vi "parseDataBoolean.vi"(8 "error in (no error)":errorcluster, 10 "Index":i32, 11 "U8ArrayParserManualIndexing in":refnum<class "U8ArrayParserManualIndexing.lvclass">) -> (0 "error out":errorcluster, 1 "Data":bool, 2 "Index out":i32, 3 "U8ArrayParserManualIndexing out":refnum<class "U8ArrayParserManualIndexing.lvclass">)   [LabVIEW 2016, in "RTUtilities.lvlib" / "U8ArrayParserManualIndexing.lvclass"]
uses:
  U8ArrayParserManualIndexing.lvclass
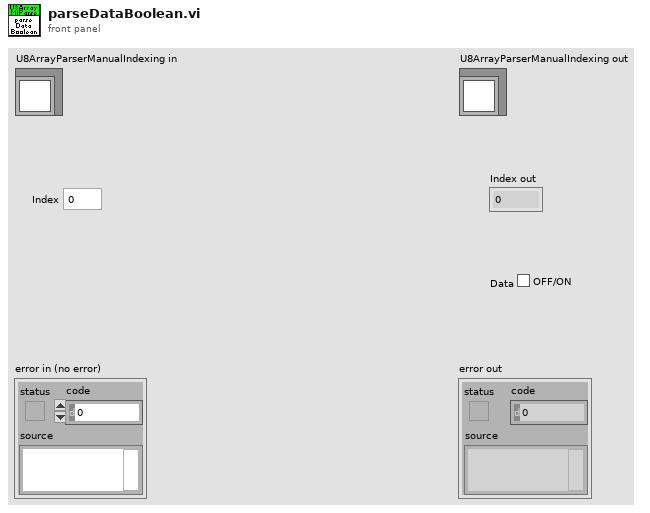
[diagram p1: front panel]
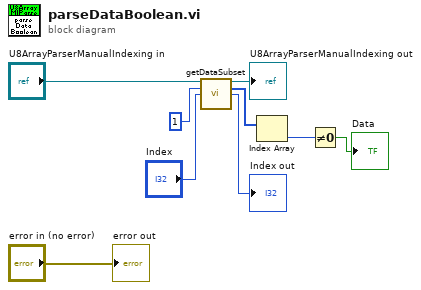
[diagram p0: block diagram]
diagram:
  n1 = call "getDataSubset.vi"("U8ArrayParserManualIndexing in"="U8ArrayParserManualIndexing in", "Length"=1, "Index"="Index") -> ("U8ArrayParserManualIndexing out"=→"U8ArrayParserManualIndexing out":refnum<class "U8ArrayParserManualIndexing.lvclass">, "Data"=w3:u8[], "Index out"=→"Index out":i32)  [unwired: 9 in, 1 out]
  n2 = Index Array(array=w3) -> (element=w2:u8)  [unwired: 1 in]
  n3 = Not Equal To 0?(x=w2) -> (x != 0?=→"Data":bool)
  "error out" <- "error in (no error)"
